vi "Division (SubVI).vi"(10 "Numeric #2":dbl, 11 "Numeric #1":dbl) -> (3 "Numeric":dbl)   [LabVIEW 2017]
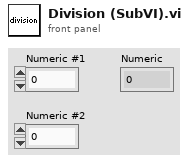
[diagram p1: front panel]
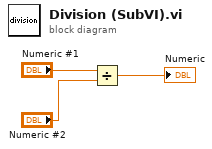
[diagram p0: block diagram]
diagram:
  n1 = Divide(x="Numeric #1", y="Numeric #2") -> (x/y=→"Numeric":dbl)
